vi "Query TX labels for Params.vi"(8 "error in":errorcluster, 11 "node result array":refnum<k20>[](array[refnum])) -> (0 "error out":errorcluster, 3 "LabelParams":T1[](array[typedef]))   [LabVIEW 2016]
uses:
  Controls/LabelParam.ctl
  Controls/LabelInfo.ctl
  Controls/ARINCParam.ctl
  <vilib>/xml/Close Reference(Node).vi
  <vilib>/xml/Close Reference(NNMap).vi
  Ballard Arinc-429 System Explorer.lvlib
  <resource>/objmgr/DOMUserDefRef.rc
  <vilib>/xml/NI_XML.lvlib
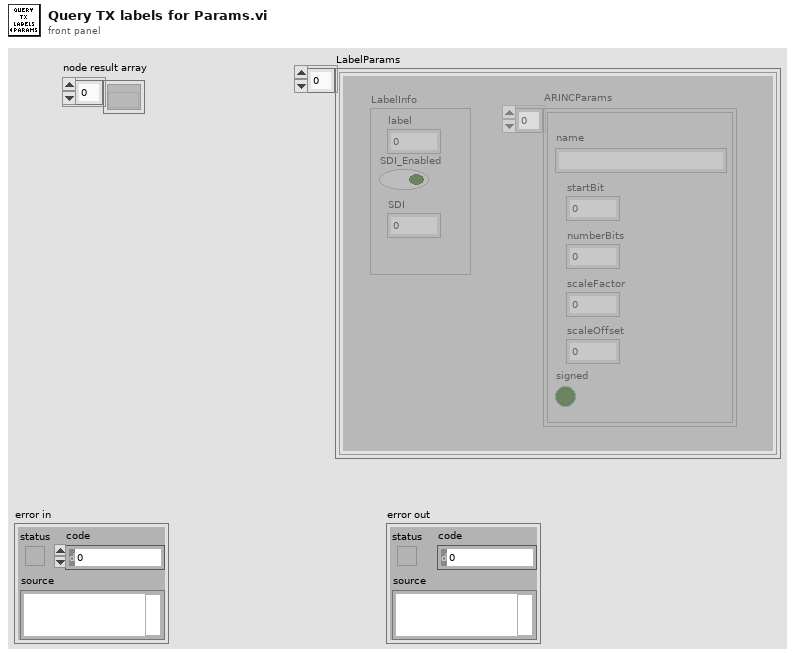
[diagram p1: front panel]
types:
  T1 = typedef "Ballard Arinc-429 System Explorer.lvlib/LabelParam.ctl" = cluster{"LabelInfo":T2, "ARINCParams":T3[]}
  T2 = typedef "Ballard Arinc-429 System Explorer.lvlib/LabelInfo.ctl" = cluster{"label":u32, "SDI_Enabled":bool, "SDI":u8}
  T3 = typedef "Ballard Arinc-429 System Explorer.lvlib/ARINCParam.ctl" = cluster{"name":string, "startBit":i32, "numberBits":i32, "scaleFactor":dbl, "scaleOffset":dbl, "signed":bool}
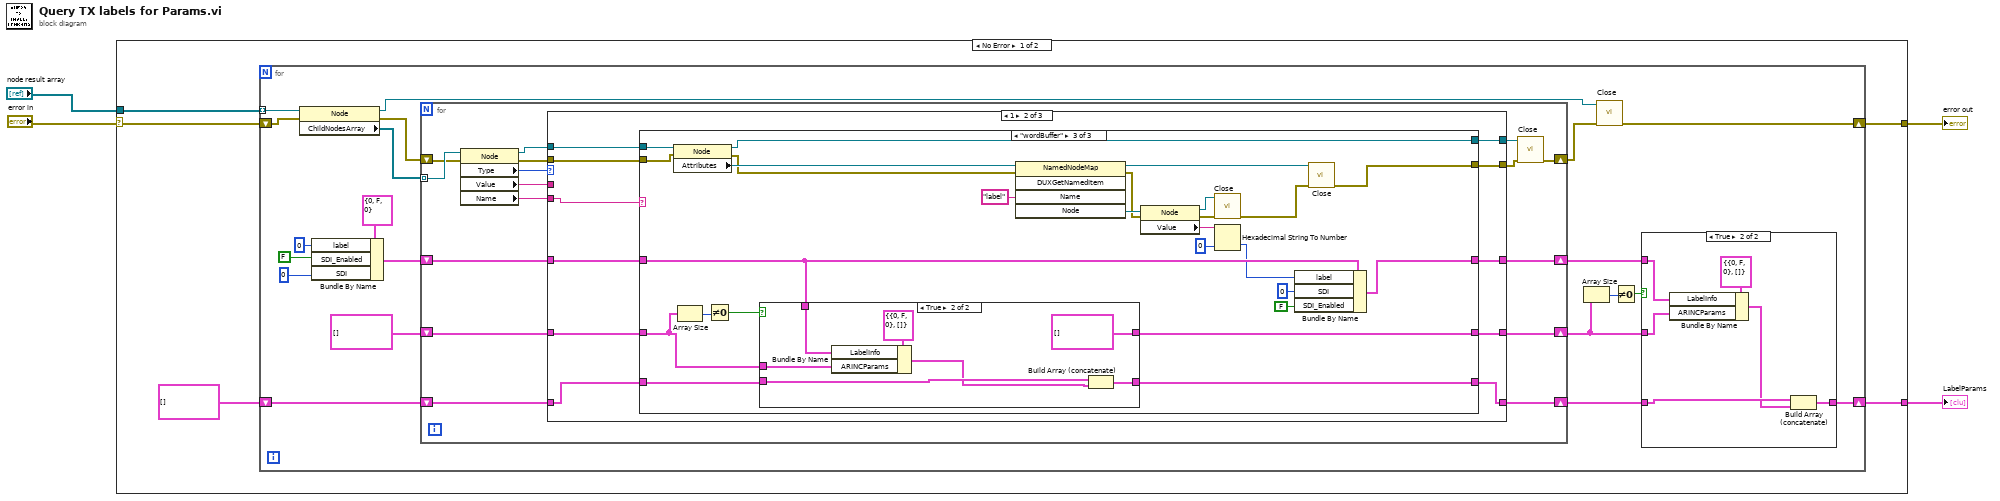
[diagram p0: block diagram]
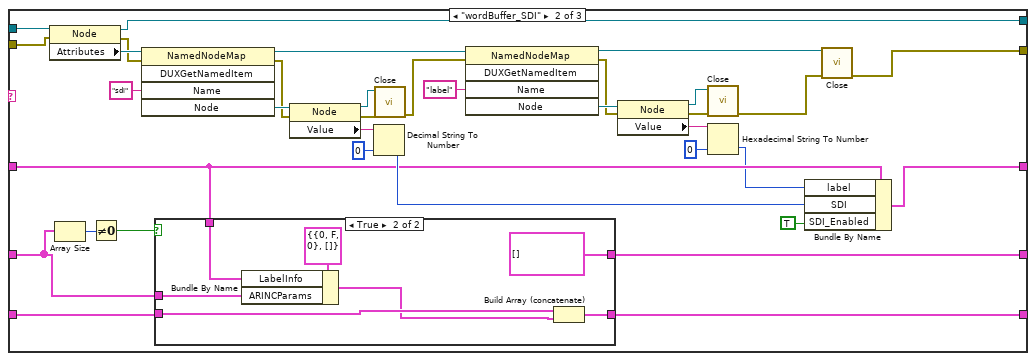
[diagram p5: hidden frame]
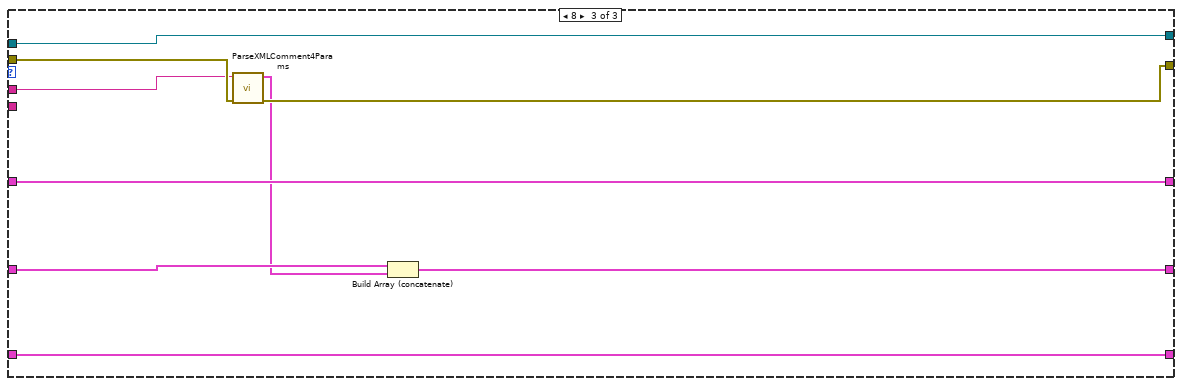
[diagram p8: hidden frame]
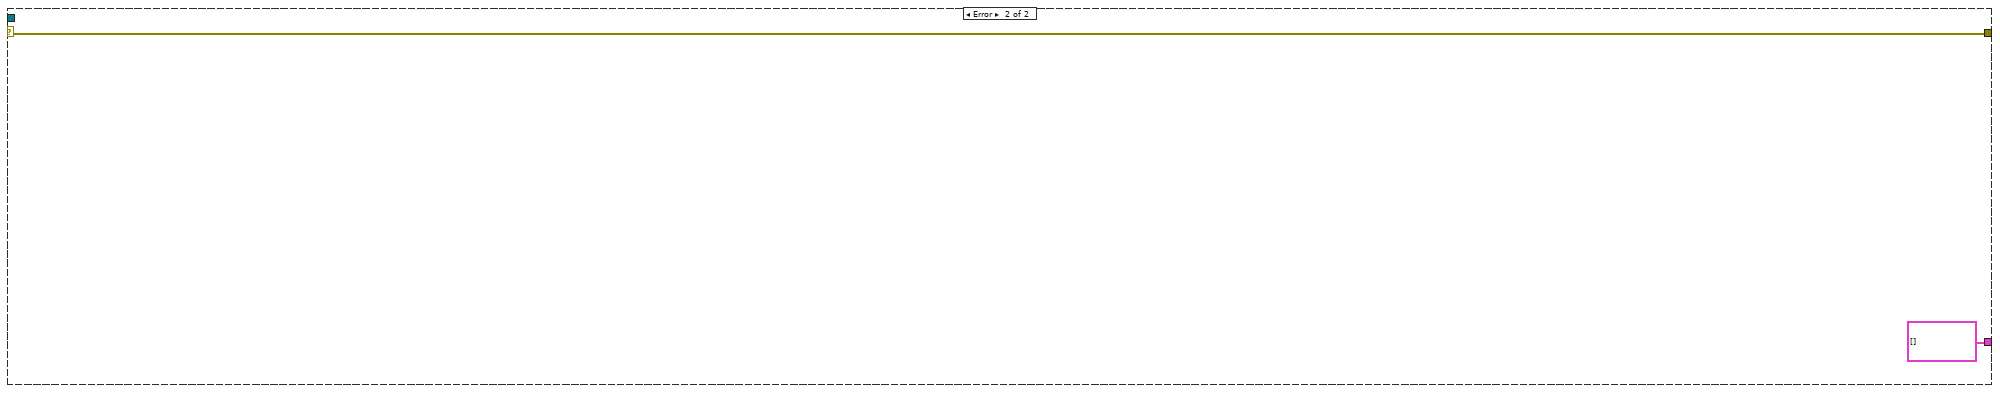
[diagram p9: hidden frame]
diagram:
  n1 = case shown="No Error" "error in" {
    selector: "error in" -> [w5 w163]
    tunnel: "node result array" -> [w8 _]
    tunnel: [w7 T1[] []] -> w1
    tunnel: [w6 w163] -> w4
    frame No Error {
      n2 = for {
        tunnel: w8 -> [w12] mode=indexing
        shift-right: [w27] -> w6
        shift-left: w5 -> [w11]
        shift-right: [w10] -> w7
        shift-left: T1[] [] -> [w20]
        n3 = property class="Node"(reference=w12, error in=w11) -> (reference out=w26:refnum<k20>, error out=w28:errorcluster, "ChildNodesArray"=w29:refnum<k20>[])
        n4 = Bundle By Name(cluster=T2 {"label"=0, "SDI_Enabled"=FALSE, "SDI"=0} ("output cluster"), "label"=u32 0, "SDI_Enabled"=FALSE, "SDI"=u8 0 ("default (0 I32)")) -> (w22:T2)
        n5 = for {
          tunnel: w29 -> [w52] mode=indexing
          shift-right: [w47] -> w25
          shift-left: w28 -> [w51]
          shift-right: [w42] -> w14
          shift-left: w22 -> [w43]
          shift-right: [w40] -> w15
          shift-left: w20 -> [w41]
          shift-right: [w38] -> w16
          shift-left: T3[] [] -> [w39]
          n6 = property class="Node"(reference=w52, error in=w51) -> (reference out=w45:refnum<k20>, error out=w48:errorcluster, "Type"=w50:i32, "Value"=w49:string, "Name"=w37:string)
          n7 = case shown="1" w50 {
            tunnel: w49 -> [_ _ w160]
            tunnel: w48 -> [w57 w66 w161]
            tunnel: [w57 w65 w159] -> w46
            tunnel: w45 -> [w54 w68 w158]
            tunnel: [w54 w67 w158] -> w44
            tunnel: w43 -> [w56 w61 w157]
            tunnel: [w56 w64 w157] -> w42
            tunnel: w41 -> [w55 w63 w153]
            tunnel: [w55 w62 w153] -> w40
            tunnel: w39 -> [w53 w60 w156]
            tunnel: [w53 w59 w154] -> w38
            tunnel: w37 -> [_ w58 _]
            frame 0, Default {
            }
            frame 1 {
              n8 = case shown="\"wordBuffer\"" w58 {
                tunnel: w68 -> [w69 w108 w143]
                tunnel: [w69 w107 w142] -> w67
                tunnel: w66 -> [w70 w106 w141]
                tunnel: [w70 w98 w140] -> w65
                tunnel: [w73 w93 w138] -> w64
                tunnel: w63 -> [w71 w90 w135]
                tunnel: [w71 w89 w134] -> w62
                tunnel: w61 -> [w73 w88 w133]
                tunnel: w60 -> [w72 w87 w132]
                tunnel: [w72 w86 w131] -> w59
                frame "", Default {
                }
                frame "wordBuffer_SDI" {
                  n9 = property class="Node"(reference=w108, error in=w106) -> (reference out=w107:refnum<k20>, error out=w103:errorcluster, "Attributes"=w105:refnum<k20>)
                  n10 = Array Size(array=w87) -> (size(s)=w92:i32)
                  n11 = Not Equal To 0?(x=w92) -> (x != 0?=w91:bool)
                  n12 = invoke class="NamedNodeMap" method="DUXGetNamedItem"(reference=w105, error in=w103, "Name"="sdi") -> (reference out=w85:refnum<k20>, error out=w101:errorcluster, "Node"=w102:refnum<k20>)  [unwired: 2 in, 2 out]
                  n13 = case shown="True" w91 {
                    tunnel: w90 -> [w110 w117]
                    tunnel: [w110 w116] -> w89
                    tunnel: w88 -> [_ w113]
                    tunnel: w87 -> [w109 w112]
                    tunnel: [w109 T3[] []] -> w86
                    frame False {
                    }
                    frame True {
                      n14 = Bundle By Name(cluster=T1 {"LabelInfo"={"label"=0, "SDI_Enabled"=FALSE, "SDI"=0}, "ARINCParams"=[]} ("LabelParam"), "LabelInfo"=w113, "ARINCParams"=w112) -> (w114:T1)
                      n15 = Build Array (concatenate)(w117, w114) -> (w116:T1[])
                    }
                  }
                  n16 = property class="Node"(reference=w102, error in=w101) -> (reference out=w99:refnum<k20>, error out=w100:errorcluster, "Value"=w94:string)
                  n17 = Decimal String To Number(string=w94, default (0L)=u8 0 ("default (0 I32)")) -> (number=w97:u8)  [unwired: 1 in, 1 out]
                  n18 = call-poly <vilib>:"Close.vi"("error in (no error)"=w100, "node"=w99) -> ("error out"=w84:errorcluster)  [unwired: 7 out]
                  n19 = invoke class="NamedNodeMap" method="DUXGetNamedItem"(reference=w85, error in=w84, "Name"="label") -> (reference out=w80:refnum<k20>, error out=w81:errorcluster, "Node"=w82:refnum<k20>)  [unwired: 2 in, 2 out]
                  n20 = property class="Node"(reference=w82, error in=w81) -> (reference out=w77:refnum<k20>, error out=w76:errorcluster, "Value"=w79:string)
                  n21 = call-poly <vilib>:"Close.vi"("error in (no error)"=w76, "node"=w77) -> ("error out"=w75:errorcluster)  [unwired: 7 out]
                  n22 = Hexadecimal String To Number(string=w79, default (0uL)=u32 0 ("default (0 I32)")) -> (number=w74:u32)  [unwired: 1 in, 1 out]
                  n23 = Bundle By Name(cluster=w88, "label"=w74, "SDI"=w97, "SDI_Enabled"=TRUE) -> (w93:T2)
                  n24 = call-poly <vilib>:"Close.vi"("error in (no error)"=w75, "named node map"=w80) -> ("error out"=w98:errorcluster)  [unwired: 7 out]
                }
                frame "wordBuffer" {
                  n25 = property class="Node"(reference=w143, error in=w141) -> (reference out=w142:refnum<k20>, error out=w119:errorcluster, "Attributes"=w120:refnum<k20>)
                  n26 = Array Size(array=w132) -> (size(s)=w137:i32)
                  n27 = Not Equal To 0?(x=w137) -> (x != 0?=w136:bool)
                  n28 = case shown="True" w136 {
                    tunnel: w135 -> [w145 w152]
                    tunnel: [w145 w151] -> w134
                    tunnel: w133 -> [_ w148]
                    tunnel: w132 -> [w144 w147]
                    tunnel: [w144 T3[] []] -> w131
                    frame False {
                    }
                    frame True {
                      n29 = Bundle By Name(cluster=T1 {"LabelInfo"={"label"=0, "SDI_Enabled"=FALSE, "SDI"=0}, "ARINCParams"=[]} ("LabelParam"), "LabelInfo"=w148, "ARINCParams"=w147) -> (w149:T1)
                      n30 = Build Array (concatenate)(w152, w149) -> (w151:T1[])
                    }
                  }
                  n31 = invoke class="NamedNodeMap" method="DUXGetNamedItem"(reference=w120, error in=w119, "Name"="label") -> (reference out=w127:refnum<k20>, error out=w128:errorcluster, "Node"=w129:refnum<k20>)  [unwired: 2 in, 2 out]
                  n32 = property class="Node"(reference=w129, error in=w128) -> (reference out=w124:refnum<k20>, error out=w123:errorcluster, "Value"=w126:string)
                  n33 = call-poly <vilib>:"Close.vi"("error in (no error)"=w123, "node"=w124) -> ("error out"=w122:errorcluster)  [unwired: 7 out]
                  n34 = Hexadecimal String To Number(string=w126, default (0uL)=u32 0 ("default (0 I32)")) -> (number=w121:u32)  [unwired: 1 in, 1 out]
                  n35 = Bundle By Name(cluster=w133, "label"=w121, "SDI"=u8 0, "SDI_Enabled"=FALSE) -> (w138:T2)
                  n36 = call-poly <vilib>:"Close.vi"("error in (no error)"=w122, "named node map"=w127) -> ("error out"=w140:errorcluster)  [unwired: 7 out]
                }
              }
            }
            frame 8 {
              n37 = call "ParseXMLComment4Params.vi"("error in"=w161, "XML Comment"=w160) -> ("error out"=w159:errorcluster, "ARINC Parameter"=w155:T3)  [unwired: 8 in]
              n38 = Build Array (concatenate)(w156, w155) -> (w154:T3[])
            }
          }
          n39 = call-poly <vilib>:"Close.vi"("error in (no error)"=w46, "node"=w44) -> ("error out"=w47:errorcluster)  [unwired: 7 out]
        }
        n40 = Array Size(array=w16) -> (size(s)=w18:i32)
        n41 = call-poly <vilib>:"Close.vi"("error in (no error)"=w25, "node"=w26) -> ("error out"=w27:errorcluster)  [unwired: 7 out]
        n42 = Not Equal To 0?(x=w18) -> (x != 0?=w17:bool)
        n43 = case shown="True" w17 {
          tunnel: w16 -> [_ w31]
          tunnel: w15 -> [w30 w33]
          tunnel: [w30 w34] -> w10
          tunnel: w14 -> [_ w35]
          frame False {
          }
          frame True {
            n44 = Bundle By Name(cluster=T1 {"LabelInfo"={"label"=0, "SDI_Enabled"=FALSE, "SDI"=0}, "ARINCParams"=[]} ("LabelParam"), "LabelInfo"=w35, "ARINCParams"=w31) -> (w32:T1)
            n45 = Build Array (concatenate)(w33, w32) -> (w34:T1[])
          }
        }
      }
    }
    frame Error {
    }
  }
  "LabelParams" <- w1
  "error out" <- w4
